vi "dialog save dirty dot.vi"(8 "error in":errorcluster, 9 "View":refnum<vi>, 11 "state in":T1) -> (0 "error out":errorcluster, 1 "new":bool, 3 "state out":T1)   [LabVIEW 2013, in "Standard Editor.lvlib"]
uses:
  Standard Editor.lvlib
  Controls/StateCluster.ctl
  Configuration Editor/Classes/SystemConfigRepo/SystemConfigRepo.lvclass
  Configuration Editor/Classes/Systems/Systems.lvclass
  <vilib>/NI/Configuration Framework/Node/StandardEvents.ctl
  <vilib>/NI/Configuration Framework/Node/UserEventRef.ctl
  <vilib>/NI/Configuration Framework/Controls/EventCluster.ctl
  <vilib>/NI/Configuration Framework/Node/NodeChangeEvent.ctl
  <vilib>/NI/Configuration Framework/Node/NodeRef.ctl
  <vilib>/NI/Configuration Framework/Node/NISE_CEF_Node.lvclass
  <vilib>/NI/Configuration Framework/Node/CacheState.ctl
  <vilib>/NI/Configuration Framework/Node/RefreshUIEvent.ctl
  <vilib>/NI/Configuration Framework/Node/StopEvent.ctl
  <vilib>/NI/Configuration Framework/glyph manager/glyph manager.ctl
  <vilib>/picture/picture.llb/imagedata.ctl
  <vilib>/NI/AMC/Message Queue.ctl
  <vilib>/NI/AMC/Message.ctl
  <vilib>/NI/Tools/Keyed Array/KeyedArray.ctl
  <vilib>/NI/Configuration Framework/NISE_CEF_TreeControl.lvlib
  <vilib>/NI/Configuration Framework/glyph manager/glyph manager.lvlib
  <vilib>/NI/Tools/Keyed Array/Tools_KeyedArray.lvlib
  <vilib>/NI/AMC/AMC.lvlib
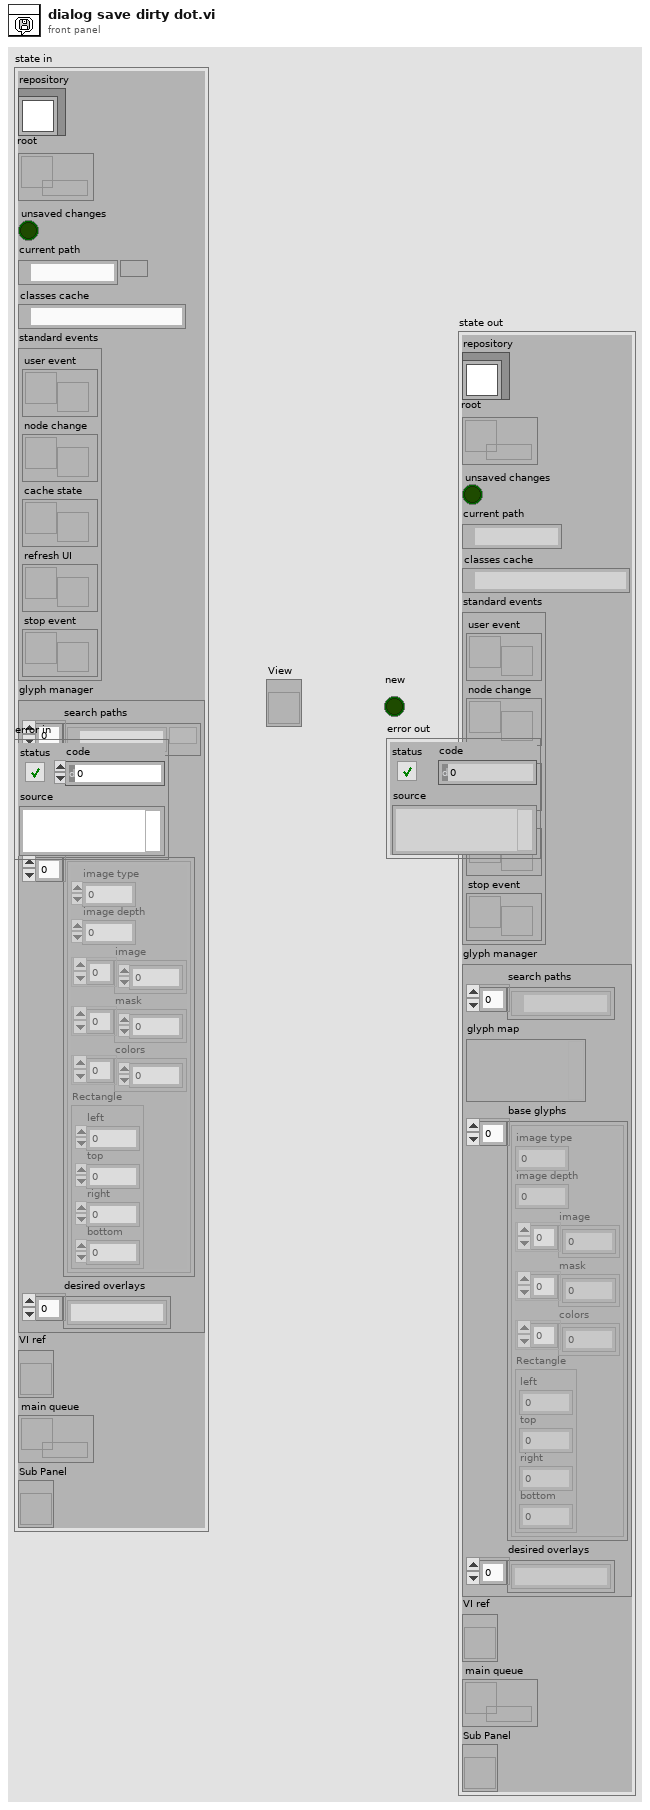
[diagram p1: front panel]
types:
  T1 = typedef "Standard Editor.lvlib/StateCluster.ctl" = cluster{"repository":refnum<class "SystemConfigRepo.lvclass">, "root":refnum<data-value>, "unsaved changes":bool, "current path":path, "classes cache":path, "standard events":T2, "glyph manager":T8, "VI ref":refnum<vi>, "main queue":T10, "Sub Panel":refnum<vi>}
  T2 = typedef "NISE_CEF_Node.lvclass/StandardEvents.ctl" = cluster{"user event":T3, "node change":T4, "cache state":T5, "refresh UI":T6, "stop event":T7}
  T3 = typedef "NISE_CEF_Node.lvclass/UserEventRef.ctl" = refnum<user-event>
  T4 = typedef "NISE_CEF_Node.lvclass/NodeChangeEvent.ctl" = refnum<user-event>
  T5 = typedef "NISE_CEF_Node.lvclass/CacheState.ctl" = refnum<user-event>
  T6 = typedef "NISE_CEF_Node.lvclass/RefreshUIEvent.ctl" = refnum<user-event>
  T7 = typedef "NISE_CEF_Node.lvclass/StopEvent.ctl" = refnum<user-event>
  T8 = typedef "glyph manager.lvlib/glyph manager.ctl" = cluster{"search paths":path[], "glyph map":variant, "base glyphs":T9[], "desired overlays":string[]}
  T9 = typedef "imagedata.ctl" = cluster{"image type":i32, "image depth":i32, "image":u8[], "mask":u8[], "colors":u32[], "Rectangle":cluster{"left":i16, "top":i16, "right":i16, "bottom":i16}}
  T10 = typedef "AMC.lvlib/Message Queue.ctl" = refnum<queue>
  T11 = enum16{"Left Button", "Center Button", "Right Button", "Window Close"}
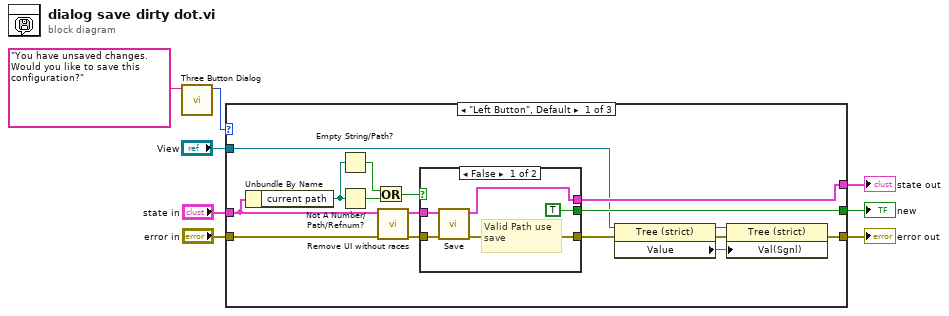
[diagram p0: block diagram]
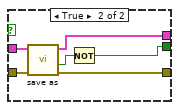
[diagram p2: hidden frame]
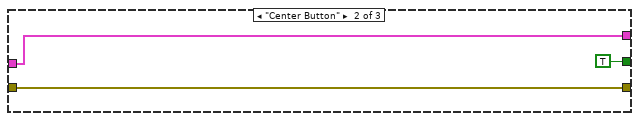
[diagram p3: hidden frame]
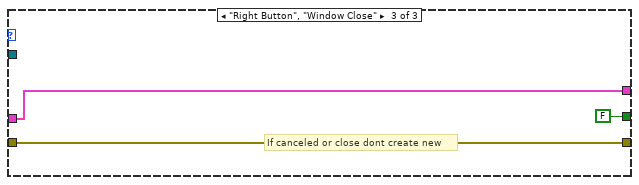
[diagram p4: hidden frame]
diagram:
  n1 = call <vilib>:"Three Button Dialog.vi"("message"="You have unsaved changes.  Would you like to save this configuration?") -> ("Which Button?"=w3:T11)  [unwired: 10 in]
  n2 = case shown="\"Left Button\", Default" w3 {
    tunnel: "state in" -> [w10 w37 w40]
    tunnel: [w20 w37 w40] -> w7
    tunnel: "error in" -> [w18 w36 w39]
    tunnel: [w13 w36 w39] -> w5
    tunnel: [w19 TRUE ("New") FALSE ("New")] -> w2
    tunnel: "View" -> [w12 _ _]
    frame "Left Button", Default {
      n3 = Unbundle By Name(w10) -> ("current path"=w24:path)
      n4 = Empty String/Path?(string/path=w24) -> (empty?=w22:bool)
      n5 = Not A Number/Path/Refnum?(number/path/refnum=w24) -> (NaN/Path/Refnum?=w21:bool)
      n6 = Or(x=w22, y=w21) -> (x .or. y?=w23:bool)
      n7 = call "Remove UI without races.vi"("error in"=w18, "state in"=w10) -> ("error out"=w17:errorcluster, "state out"=w9:T1)  [unwired: 8 in]
      n8 = case shown="False" w23 {
        tunnel: w9 -> [w26 w33]
        tunnel: [w29 w32] -> w20
        tunnel: [w25 w34] -> w14
        tunnel: w17 -> [w27 w35]
        tunnel: [TRUE w30] -> w19
        frame False {
          # "Valid Path use save"
          n9 = call "Save.vi"("error in"=w27, "state in"=w26) -> ("error out"=w25:errorcluster, "state out"=w29:T1)  [unwired: 8 in]
        }
        frame True {
          n10 = call "save as.vi"("error in"=w35, "state in"=w33) -> ("error out"=w34:errorcluster, "canceled?"=w31:bool, "state out"=w32:T1)  [unwired: 7 in]
          n11 = Not(x=w31) -> (.not. x?=w30:bool)
        }
      }
      n12 = property class="Tree (strict)"(reference=w12, error in=w14) -> (reference out=w11:refnum<vi>, error out=w16:errorcluster, "Value"=w15:string)
      n13 = property class="Tree (strict)"(reference=w11, error in=w16, "Val(Sgnl)"=w15) -> (error out=w13:errorcluster)  [unwired: 1 out]
    }
    frame "Center Button" {
    }
    frame "Right Button", "Window Close" {
      # "If canceled or close dont create new"
    }
  }
  "state out" <- w7
  "error out" <- w5
  "new" <- w2
